vi "Configure.vi"(8 "error in":errorcluster, 10 "name":string, 11 "Instrument in":refnum<class "Instrument.lvclass">) -> (0 "error out":errorcluster, 3 "Instrument out":refnum<class "Instrument.lvclass">)   [LabVIEW 2018, in "Instrument.lvclass"]
doc: "Configure the instrument class. If there is no config file specified, an error"
uses:
  Instrument.lvclass
  Instrument.lvclass/Instrument.ctl
  Session APIs/Session Log/System Log.lvclass
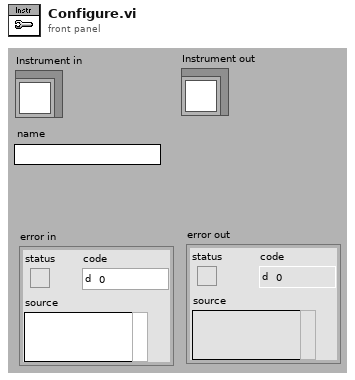
[diagram p1: front panel]
types:
  T1 = typedef "Session - Root.lvclass/Session Handle.ctl" = refnum<data-value>
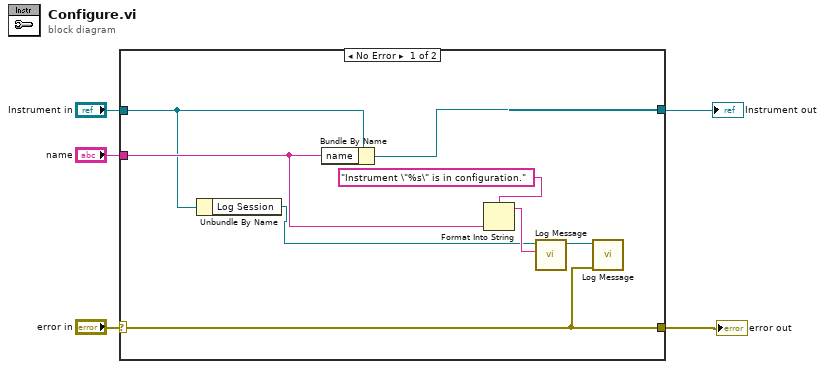
[diagram p0: block diagram]
diagram:
  n1 = case shown="No Error" "error in" {
    selector: "error in" -> [w8 w15]
    tunnel: [w8 w15] -> w4
    tunnel: [w13 w14] -> w2
    tunnel: "Instrument in" -> [w7 w14]
    tunnel: "name" -> [w9 _]
    frame No Error {
      n2 = Unbundle By Name(w7) -> ("Log Session"=w6:T1)
      n3 = Bundle By Name(cluster=w7, "name"=w9) -> (w13:refnum<class "Instrument.lvclass">)
      n4 = Format Into String(format string="Instrument \"%s\" is in configuration.", w9) -> (resulting string=w11:string)  [unwired: 2 in, 1 out]
      n5 = call "Log Message.vi"("MSG In"=w11, "session in"=w6) -> ("session out"=w12:T1)  [unwired: 8 in, 1 out]
      n6 = call "Log Message.vi"("error in"=w8, "session in"=w12) -> ()  [unwired: 8 in, 2 out]
    }
    frame Error {
    }
  }
  "error out" <- w4
  "Instrument out" <- w2
